vi "ExecuteVI.vi"(5 "CmdData":variant, 6 "HighPrio":bool, 7 "CmdVIRef":refnum<vi>, 8 "ErrorIn":errorcluster, 9 "VIToExecute":refnum<vi>, 10 "Name":string, 11 "YActorIn":refnum<class "YActor.lvclass">) -> (0 "ErrorOut":errorcluster, 2 "ReplyData":variant, 3 "YActorOut":refnum<class "YActor.lvclass">)   [LabVIEW 2021, in "YActor.lvclass"]
uses:
  YActor.lvclass
  YActor.lvclass/YActor.ctl
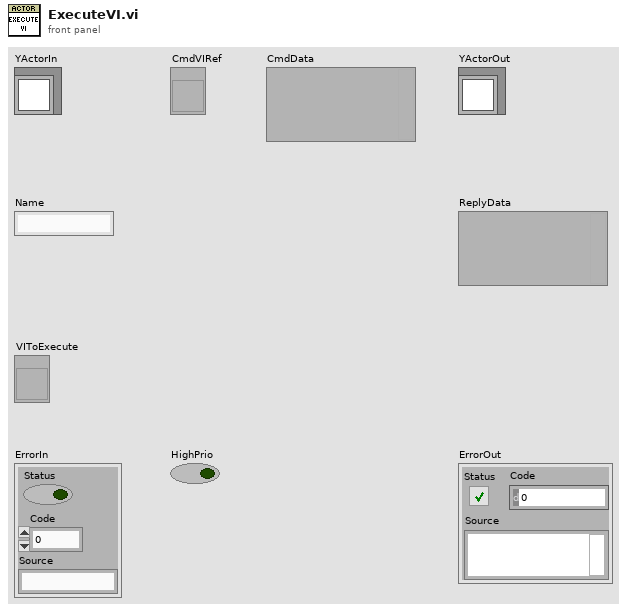
[diagram p1: front panel]
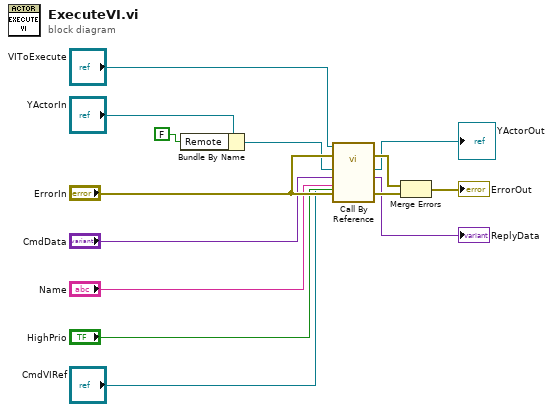
[diagram p0: block diagram]
diagram:
  n1 = Bundle By Name(cluster="YActorIn", "Remote"=FALSE ("Remote.Remote?")) -> (w2:refnum<class "YActor.lvclass">)
  n2 = call-by-ref "?"(reference="VIToExecute", error in="ErrorIn", "HighPrio"="HighPrio", "CmdVIRef"="CmdVIRef", "ErrorIn"="ErrorIn", "NameOfVi2Call(optional)"="Name", "CmdData"="CmdData", "ReferenceIn"=w2) -> (error out=w12:errorcluster, "ErrorOut"=w13:errorcluster, "ReplyData"=→"ReplyData":variant, "ReferenceOut"=→"YActorOut":refnum<class "YActor.lvclass">)  [unwired: 3 in, 1 out]
  n3 = Merge Errors(w12, w13) -> (→"ErrorOut":errorcluster)
